vi "ex7_shift register.vi"() -> ()   [LabVIEW 2018]
panel:
  out "Numeric 2":dbl
  in  "stop":bool
  out "Numeric":dbl
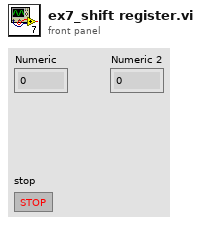
[diagram p1: front panel]
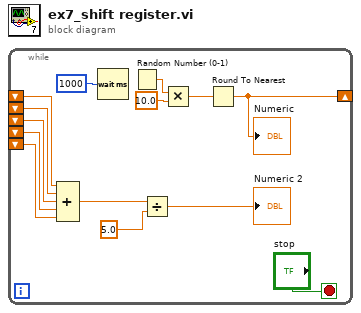
[diagram p0: block diagram]
diagram:
  n1 = while {
    shift-right: [w9] -> _
    shift-left: _ -> [w8]
    shift-left: _ -> [w7]
    shift-left: _ -> [w6]
    shift-left: _ -> [w5]
    shift-left: _ -> [w4]
    stop <- "stop" stop-if-true
    n2 = Compound Arithmetic op=ADD(w8, w7, w6, w5, w4) -> (w2:dbl)
    n3 = Wait (ms)(milliseconds to wait=u32 1000 ("millisecond timer value")) -> ()  [unwired: 1 out]
    n4 = Random Number (0-1)() -> (number: 0 to 1=w13:dbl)
    n5 = Divide(x=w2, y=5.0) -> (x/y=→"Numeric 2":dbl)
    n6 = Multiply(x=w13, y=10.0) -> (x*y=w14:dbl)
    n7 = Round To Nearest(number=w14) -> (nearest integer value=w9:dbl)
    "Numeric" <- w9
  }
